vi "Get WhileLoop Terminals.vi"(8 "error in":errorcluster, 11 "reference":refnum<vi>) -> (0 "error out":errorcluster, 3 "tunnel refs.":refnum<vi>[](array[refnum]))   [LabVIEW 2014]
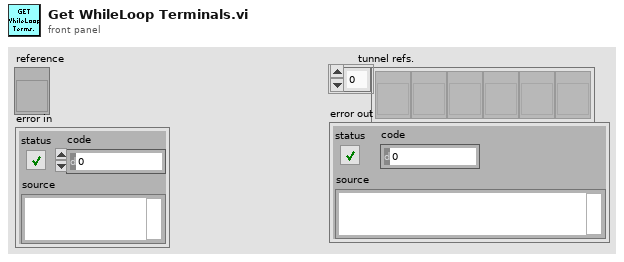
[diagram p1: front panel]
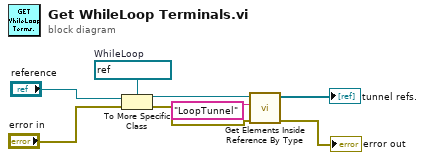
[diagram p0: block diagram]
diagram:
  w4 = refnum<vi> refnum  # WhileLoop
  n1 = To More Specific Class(target class=w4, reference="reference", error in="error in") -> (specific class reference=w7:refnum<vi>, error out=w2:errorcluster)
  n2 = call "Get Elements Inside Reference By Type.vi"("error in (no error)"=w2, "filter element class name"="LoopTunnel", "element ref."=w7) -> ("error out"=→"error out":errorcluster, "elements ref."=→"tunnel refs.":refnum<vi>[])  [unwired: 6 in, 1 out]
